vi "CalibrateTANGO.vi"(8 "error in (no error)":errorcluster, 11 "plLSID in":i32) -> (0 "error out":errorcluster, 2 "X Limits":dbl[](array[numeric]) caption="X Limits [µm]" format="%#_10f", 3 "Y Limits":dbl[](array[numeric]) caption="Y Limits [µm]" format="%#_12f")   [LabVIEW 2018]
uses:
  <userlib>/TANGO_DLL/Tango_DLL.lvlib
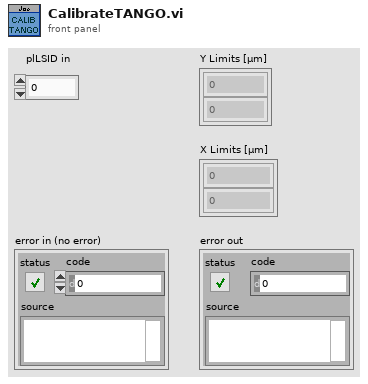
[diagram p1: front panel]
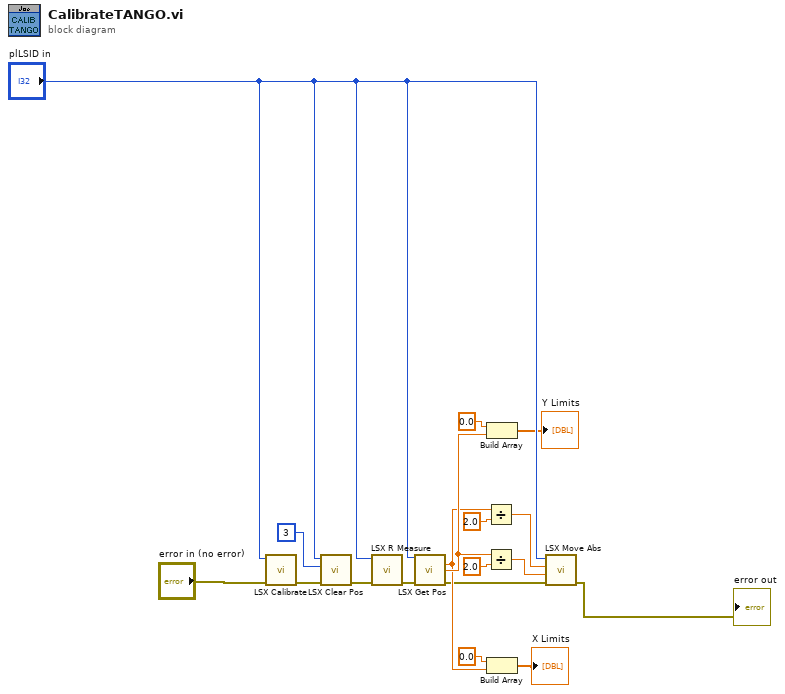
[diagram p0: block diagram]
diagram:
  n1 = call <userlib>:"LSX Calibrate.vi"("error in (no error)"="error in (no error)", "lLSID"="plLSID in") -> ("error out"=w3:errorcluster)  [unwired: 8 in, 1 out]
  n2 = call <userlib>:"LSX Clear Pos.vi"("error in (no error)"=w3, "lFlags"=i16 3, "lLSID"="plLSID in") -> ("error out"=w5:errorcluster)  [unwired: 7 in, 1 out]
  n3 = call <userlib>:"LSX R Measure.vi"("error in (no error)"=w5, "lLSID"="plLSID in") -> ("error out"=w6:errorcluster)  [unwired: 8 in, 1 out]
  n4 = call <userlib>:"LSX Get Pos.vi"("lLSID"="plLSID in", "error in (no error)"=w6) -> ("pdX out"=w14:dbl, "pdY out"=w15:dbl, "error out"=w9:errorcluster)  [unwired: 8 in, 3 out]
  n5 = Divide(x=w14, y=2.0) -> (x/y=w11:dbl)
  n6 = Divide(x=w15, y=2.0) -> (x/y=w10:dbl)
  n7 = Build Array(0.0 ("element"), w15) -> (→"Y Limits":dbl[])
  n8 = Build Array(0.0 ("element"), w14) -> (→"X Limits":dbl[])
  n9 = call <userlib>:"LSX Move Abs.vi"("error in (no error)"=w9, "dY"=w10, "dX"=w11, "lLSID"="plLSID in") -> ("error out"=→"error out":errorcluster)  [unwired: 6 in, 1 out]
